vi "Main -- video stream.vi"() -> ()   [LabVIEW 2013]
uses:
  <vilib>/userdefined/High Color/IMAQdx.ctl
  <vilib>/vision/driver/NI_Vision_Acquisition_Software.lvlib
  <vilib>/vision/NI_Vision_Development_Module.lvlib
  <resource>/objmgr/imaqdx.rc
panel:
  out "frame rate [fps]":dbl(slide) scale=0.0..30.0
  in  "video mode":u32
  in  "adjust saturation":bool
  in  "level":u32(slide) scale=0.0..255.0
  in  "processing":T1(ring)
  in  "ESC":bool
  in  "edge detector parameters":T2={"Sigma"=1.0, "HThresh"=0.9, "LThres"=0.2, "WindowSize"=9} {"LThres" min=0 max=1 format="%.2f"; "HThresh" min=0 max=1 format="%.2f"; "Sigma" min=0 max=1 format="%.2f"}
  out "processed":T3(plugin-control)
  in  "webcam":T4="cam0"
  out "source":T3(plugin-control)
  # "LED Matrix demo"
  # "Webcam demo - video stream"
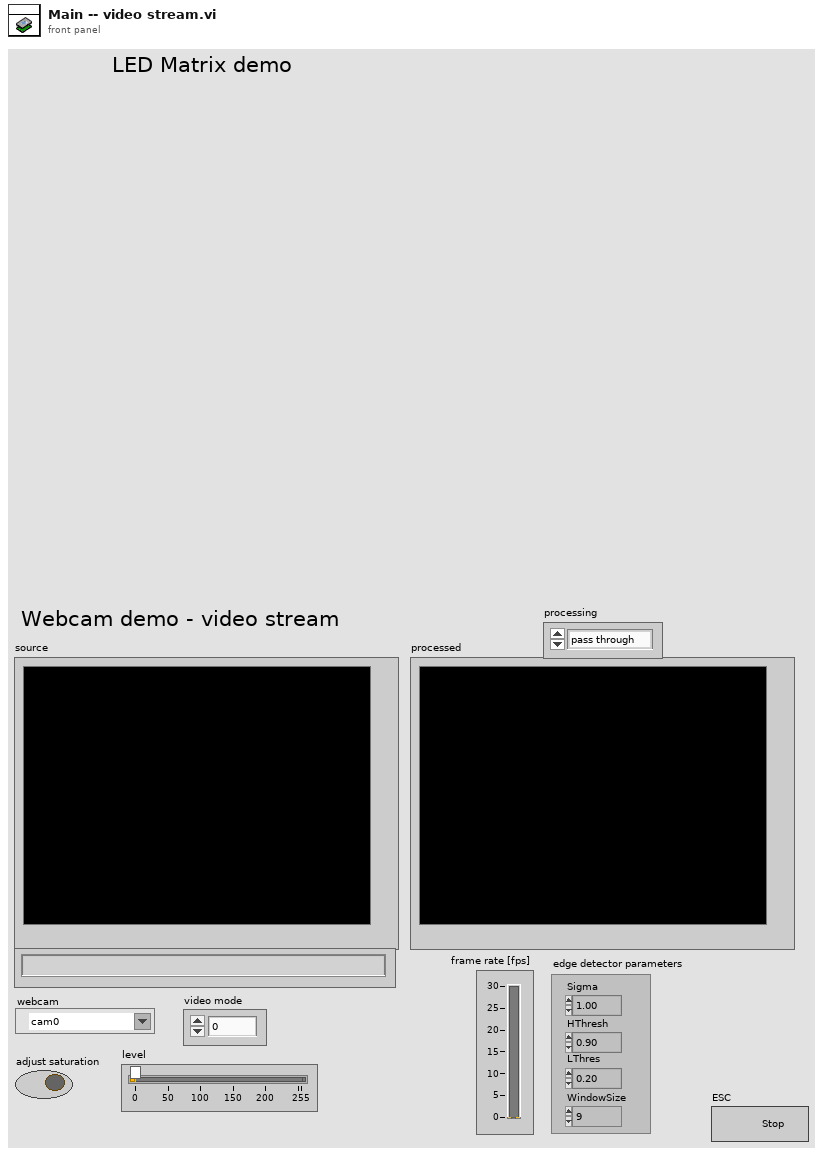
[diagram p1: front panel]
types:
  T1 = enum16{"pass through", "detect edges", "show luma", "show hue"}
  T2 = cluster{"Sigma":sgl, "HThresh":sgl, "LThres":sgl, "WindowSize":i32}
  T3 = typedef "IMAQ Image.ctl" = refnum<image>
  T4 = typedef "IMAQdx.ctl" = refnum<k21>
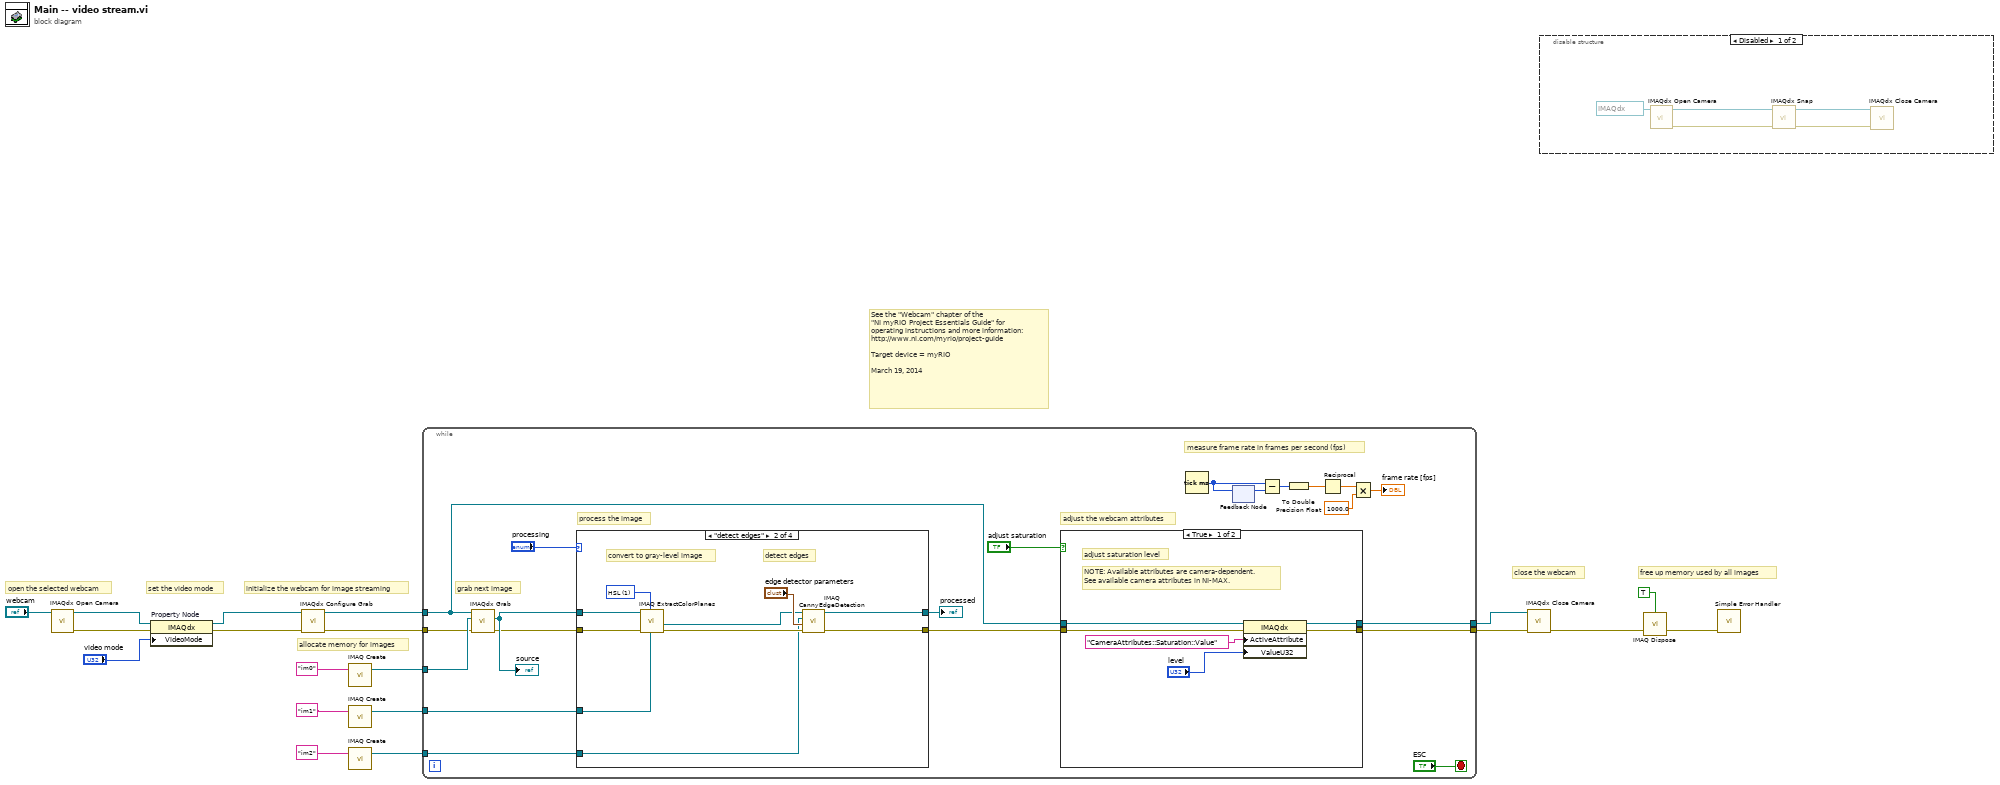
[diagram p0: block diagram]
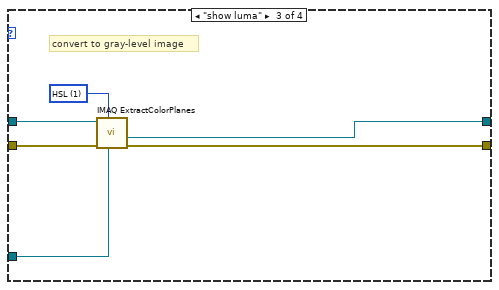
[diagram p4: hidden frame]
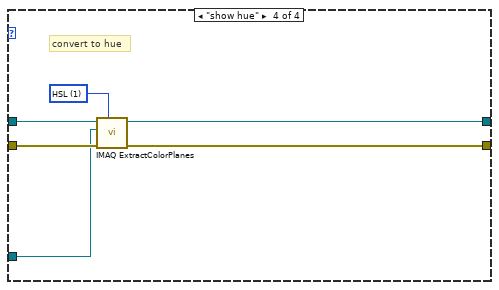
[diagram p5: hidden frame]
diagram:
  # "See the \"Webcam\" chapter of the\n\"NI myRIO Project Essentials Guide\" for\noperating instructions and more information: \nhttp://www.ni.com/myrio/project-guide\n\nTarget device = myRIO\n\nMarch 19, 2014"
  # "close the webcam"
  # "open the selected webcam"
  # "set the video mode"
  # "allocate memory for images"
  # "initialize the webcam for image streaming"
  # "free up memory used by all images"
  n1 = call <vilib>:"IMAQdx Open Camera.vi"("Session In"="webcam") -> ("error out"=w5:errorcluster, "Session Out"=w4:T4)  [unwired: 2 in, 7 out]
  n2 = property on="Property Node" class="IMAQdx"(reference=w4, error in=w5, "VideoMode"="video mode") -> (reference out=w1:T4, error out=w2:errorcluster)
  n3 = call <vilib>:"IMAQdx Configure Grab.vi"("error in"=w2, "Session In"=w1) -> ("error out"=w16:errorcluster, "Session Out"=w6:T4)  [unwired: 8 in]
  n4 = call "IMAQ Create"("Image Name"="im0") -> ("New Image"=w17:T3)  [unwired: 3 in, 2 out]
  n5 = call "IMAQ Create"("Image Name"="im1") -> ("New Image"=w13:T3)  [unwired: 3 in, 2 out]
  n6 = call "IMAQ Create"("Image Name"="im2") -> ("New Image"=w12:T3)  [unwired: 3 in, 2 out]
  n7 = while {
    tunnel: w17 -> [w40]
    tunnel: w16 -> [w38]
    tunnel: w13 -> [w37]
    tunnel: w12 -> [w36]
    tunnel: w6 -> [w28]
    tunnel: [w31] -> w9
    tunnel: [w27] -> w8
    stop <- "ESC" stop-if-true
    # "measure frame rate in frames per second (fps)"
    # "adjust the webcam attributes"
    # "process the image"
    # "grab next image"
    n8 = call <vilib>:"IMAQdx Grab.vi"("error in"=w38, "Image In"=w40, "Session In"=w28) -> ("error out"=w34:errorcluster, "Image Out"=w39:T3)  [unwired: 5 in, 2 out]
    "source" <- w39
    n9 = case shown="\"detect edges\"" "processing" {
      tunnel: w39 -> [w50 w60 w66 w72]
      tunnel: w37 -> [_ w57 w64 w68]
      tunnel: w36 -> [_ w51 _ _]
      tunnel: [w50 w54 w61 w67] -> w35
      tunnel: [w49 w53 w62 w69] -> w30
      tunnel: w34 -> [w49 w52 w63 w70]
      frame "pass through", Default {
      }
      frame "detect edges" {
        w59 = u16 1 items=["RGB", "HSL", "HSV", "HSI"] ("Color Mode")
        # "detect edges"
        # "convert to gray-level image"
        n10 = call "IMAQ ExtractColorPlanes"("Blue or Luma or Val or Inten Plane"=w57, "Color Mode"=w59, "error in (no error)"=w52, "Image Src"=w60) -> ("error out"=w56:errorcluster, "Blue or Luma or Val or Inten Plane out"=w55:T3)  [unwired: 4 in, 2 out]
        n11 = call "IMAQ CannyEdgeDetection"("Image Src"=w55, "Image Dst"=w51, "Filter Parameters"="edge detector parameters", "error in (no error)"=w56) -> ("Image Dst Out"=w54:T3, "error out"=w53:errorcluster)  [unwired: 4 in]
      }
      frame "show luma" {
        w65 = u16 1 items=["RGB", "HSL", "HSV", "HSI"] ("Color Mode")
        # "convert to gray-level image"
        n12 = call "IMAQ ExtractColorPlanes"("Blue or Luma or Val or Inten Plane"=w64, "Color Mode"=w65, "error in (no error)"=w63, "Image Src"=w66) -> ("error out"=w62:errorcluster, "Blue or Luma or Val or Inten Plane out"=w61:T3)  [unwired: 4 in, 2 out]
      }
      frame "show hue" {
        w71 = u16 1 items=["RGB", "HSL", "HSV", "HSI"] ("Color Mode")
        # "convert to hue"
        n13 = call "IMAQ ExtractColorPlanes"("Color Mode"=w71, "error in (no error)"=w70, "Red or Hue Plane"=w68, "Image Src"=w72) -> ("error out"=w69:errorcluster, "Red or Hue Plane out"=w67:T3)  [unwired: 4 in, 2 out]
      }
    }
    "processed" <- w35
    n14 = case shown="True" "adjust saturation" {
      tunnel: [w45 w48] -> w31
      tunnel: w30 -> [w41 w48]
      tunnel: w28 -> [w42 w47]
      tunnel: [w46 w47] -> w27
      frame True {
        # "NOTE: Available attributes are camera-dependent. \nSee available camera attributes in NI-MAX."
        # "adjust saturation level"
        n15 = property class="IMAQdx"(reference=w42, error in=w41, "ActiveAttribute"="CameraAttributes::Saturation::Value", "ValueU32"="level") -> (reference out=w46:T4, error out=w45:errorcluster)
      }
      frame False {
      }
    }
    n16 = Tick Count (ms)() -> (millisecond timer value=w26:u32)
    n17 = feedback-in #1(w26) -> ()
    n18 = feedback #1() -> (w25:u32)  [unwired: 1 in]
    n19 = Subtract(x=w26, y=w25) -> (x-y=w24:u32)
    n20 = To Double Precision Float(number=w24) -> (double precision float=w23:dbl)
    n21 = Reciprocal(x=w23) -> (1/x=w22:dbl)
    n22 = Multiply(x=w22, y=1000.0) -> (x*y=→"frame rate [fps]":dbl)
  }
  n23 = call <vilib>:"IMAQdx Close Camera.vi"("error in"=w9, "Session In"=w8) -> ("error out"=w10:errorcluster)  [unwired: 9 out]
  n24 = disable-structure shown="Disabled" {
    frame Disabled {
      n25 = call <vilib>:"IMAQdx Open Camera.vi"("Session In"=T4 "cam0") -> ("error out"=w76:errorcluster, "Session Out"=w75:T4)  [unwired: 9 in]
      n26 = call <vilib>:"IMAQdx Snap.vi"("error in"=w76, "Session In"=w75) -> ("error out"=w74:errorcluster, "Session Out"=w73:T4)  [unwired: 7 in, 1 out]
      n27 = call <vilib>:"IMAQdx Close Camera.vi"("error in"=w74, "Session In"=w73) -> ()  [unwired: 9 in, 1 out]
    }
    frame Enabled {
    }
  }
  n28 = call "IMAQ Dispose"("All Images? (No)"=TRUE, "error in (no error)"=w10) -> ("error out"=w7:errorcluster)  [unwired: 4 in]
  n29 = call <vilib>:"Simple Error Handler.vi"("error in (no error)"=w7) -> ()  [unwired: 4 in, 5 out]
